vi "Build Variant Request.vi"(9 "Time Stamp In":timestamp, 10 "variant in":variant, 11 "Node ID In":string) -> (3 "request out":T1 {"node status" items=["Good"=0, "Uncertain"=1073741824, "Uncertain_InitialValue"=1083310080, "Uncertain_LastUsableValue"=1083179008, "Uncertain_SensorNotAccurate"=1083375616, "Uncertain_EngineeringUnitsExceeded"=1083441152, "Bad"=2147483648, "Bad_NoCommunication"=2150694912, "Bad_NotReadable"=2151284736, "Bad_NotWritable"=2151350272, "Bad_OutOfRange"=2151415808, "Bad_WaitingForInitialData"=2150760448]})   [LabVIEW 2024]
uses:
  <vilib>/OPCUA/controls/Write Variant Request.ctl
  <vilib>/OPCUA/controls/NodeId.ctl
  <vilib>/OPCUA/controls/Write Status.ctl
panel:
  in  "request":T1 {"node status" items=["Good"=0, "Uncertain"=1073741824, "Uncertain_InitialValue"=1083310080, "Uncertain_LastUsableValue"=1083179008, "Uncertain_SensorNotAccurate"=1083375616, "Uncertain_EngineeringUnitsExceeded"=1083441152, "Bad"=2147483648, "Bad_NoCommunication"=2150694912, "Bad_NotReadable"=2151284736, "Bad_NotWritable"=2151350272, "Bad_OutOfRange"=2151415808, "Bad_WaitingForInitialData"=2150760448]}
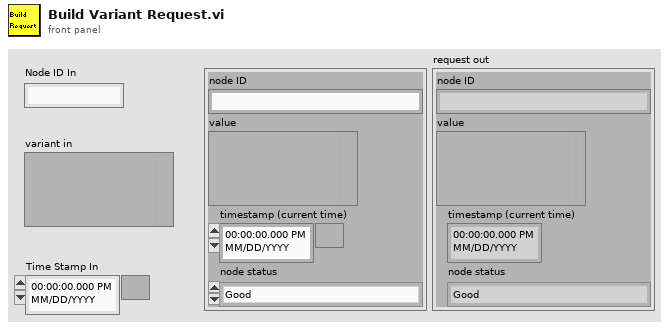
[diagram p1: front panel]
types:
  T1 = typedef "Write Variant Request.ctl" = cluster{"node ID":T2, "value":variant, "timestamp (current time)":timestamp, "node status":T3}
  T2 = typedef "NodeId.ctl" = string
  T3 = typedef "Write Status.ctl" = u32
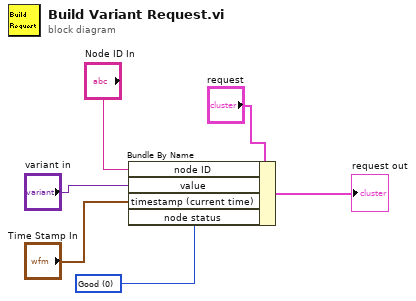
[diagram p0: block diagram]
diagram:
  w2 = T3 0 items=["Good"=0, "Uncertain"=1073741824, "Uncertain_InitialValue"=1083310080, "Uncertain_LastUsableValue"=1083179008, "Uncertain_SensorNotAccurate"=1083375616, "Uncertain_EngineeringUnitsExceeded"=1083441152, "Bad"=2147483648, "Bad_NoCommunication"=2150694912, "Bad_NotReadable"=2151284736, "Bad_NotWritable"=2151350272, "Bad_OutOfRange"=2151415808, "Bad_WaitingForInitialData"=2150760448] ("node status")
  n1 = Bundle By Name(cluster="request", "node ID"="Node ID In", "value"="variant in", "timestamp (current time)"="Time Stamp In", "node status"=w2) -> (→"request out":T1)
